vi "CG test stand DAQ main V2 variablized.vi"() -> ()   [LabVIEW 2020]
doc: "This example demonstrates how to read N channels of analog input from a LINX device."
uses:
  <vilib>/MakerHub/LINX/Public/Peripherals/Analog/Analog Read N Chans.vi
  <vilib>/MakerHub/LINX/Private/Local IO/LinxAnalogRead.vi
  <vilib>/MakerHub/LINX/Public/Utilities/Check Channel.vi
  <vilib>/MakerHub/LINX/Public/Utilities/Open Serial.vi
  <vilib>/MakerHub/LINX/Private/Utilties/Generate Error.vi
  <vilib>/Analysis/Matrix/Numeric/Conversions/Array To Matrix - RA.vi
  <vilib>/Utility/file.llb/Write Delimited Spreadsheet (DBL).vi
  <vilib>/MakerHub/LINX/LMH-LINX.lvlib
  <vilib>/Analysis/Matrix/NI_Matrix.lvlib
panel:
  in  "?":T1(tab)
  out "A8_Scaled":dbl
  out "A7_Scaled":dbl
  out "A6_Scaled":dbl
  out "C1 8":dbl
  out "C2 8":dbl
  out "C3 8":dbl
  out "B 8":dbl
  out "C1 7":dbl
  out "C2 7":dbl
  out "C3 7":dbl
  out "B 7":dbl
  out "C1 6":dbl
  out "C2 6":dbl
  out "C3 6":dbl
  out "B 6":dbl
  out "C1 5":dbl
  out "C2 5":dbl
  out "C3 5":dbl
  out "B 5":dbl
  out "C1 4":dbl
  out "C2 4":dbl
  out "C3 4":dbl
  out "B 4":dbl
  out "C1 3":dbl
  out "C2 3":dbl
  out "C3 3":dbl
  out "B 3":dbl
  out "C1 2":dbl
  out "C2 2":dbl
  out "C3 2":dbl
  out "B 2":dbl
  out "C1 1":dbl
  out "C2 1":dbl
  out "C3 1":dbl
  out "B 1":dbl
  out "C1 0":dbl
  out "C2 0":dbl
  out "C3 0":dbl
  out "B 0":dbl
  out "A0_Scaled":dbl
  out "A1_Instrumentlabel":string
  out "A8_Voltage":dbl
  out "A8":dbl
  out "A7_Voltage":dbl
  out "A7":dbl
  out "A6_Voltage":dbl
  out "A6":dbl
  out "A5_Voltage":dbl
  out "A5":dbl
  out "A4_Voltage":dbl
  out "A4":dbl
  out "A3_Voltage":dbl
  out "A3":dbl
  out "A2_Voltage":dbl
  out "A2":dbl
  out "A1_Voltage":dbl
  out "A1":dbl
  out "A0_Voltage":dbl
  out "A0_Instrumentlabel":dbl
  out "A2_Instrumentlabel":string
  out "A3_Instrumentlabel":string
  out "A4_Instrumentlabel":string
  out "A5_Instrumentlabel":string
  out "A6_Instrumentlabel":string
  out "A7_Instrumentlabel":string
  out "A8_Instrumentlabel":string
  out "A0_Instrumentlabel 2":string
  out "A1_Scaled":dbl
  out "A2_Scaled":dbl
  out "A3_Scaled":dbl
  out "A4_Scaled":dbl
  out "A5_Scaled":dbl
  in  "+      B":dbl
  in  "AX":dbl
  in  "Analog Port":dbl
  out "Time Stamp":timestamp
  out "Voltage":dbl
  out "Voltage":dbl(graph)
  out "Filtered Voltage":dbl(graph)
  out "Unfiltered Voltage":dbl
  out "Filtered Voltage":dbl
  out "?":dbl
  out "?":dbl
  out "?":dbl
  out "Orifice Temperature":dbl(knob) scale=0.0..10.0
  out "Reg Temperature":dbl(knob) scale=0.0..10.0
  out "Tank Temperature":dbl(knob) scale=0.0..10.0
  out "Temperatures":dbl[](graph)
  out "Orifice Pressure":dbl(knob) scale=0.0..10.0
  out "Reg Pressure":dbl(knob) scale=0.0..10.0
  out "Pressures":dbl[](graph)
  out "Tank Pressure":dbl(knob) scale=0.0..100.0
  in  "?":bool
  in  "Limited Rate (Hz)":dbl
  in  "?":bool
  out "Loop Rate (Hz)":u32
  in  "Stop Button":bool
  out "WRITING TO FILE":bool
  out "error out":errorcluster
  out "Full filepath":string
  in  "Path":path
  in  "File extension":string
  in  "Filename":string
  in  "Serial Port":refnum<visa-resource-name>
  # "Analog Inputs"
  # "Analog Port"
  # "Voltage In"
  # "X3"
  # "X2"
  # "X1"
  # "B"
  # "Instrument name"
  # "Scaled Value"
  # "File I/O"
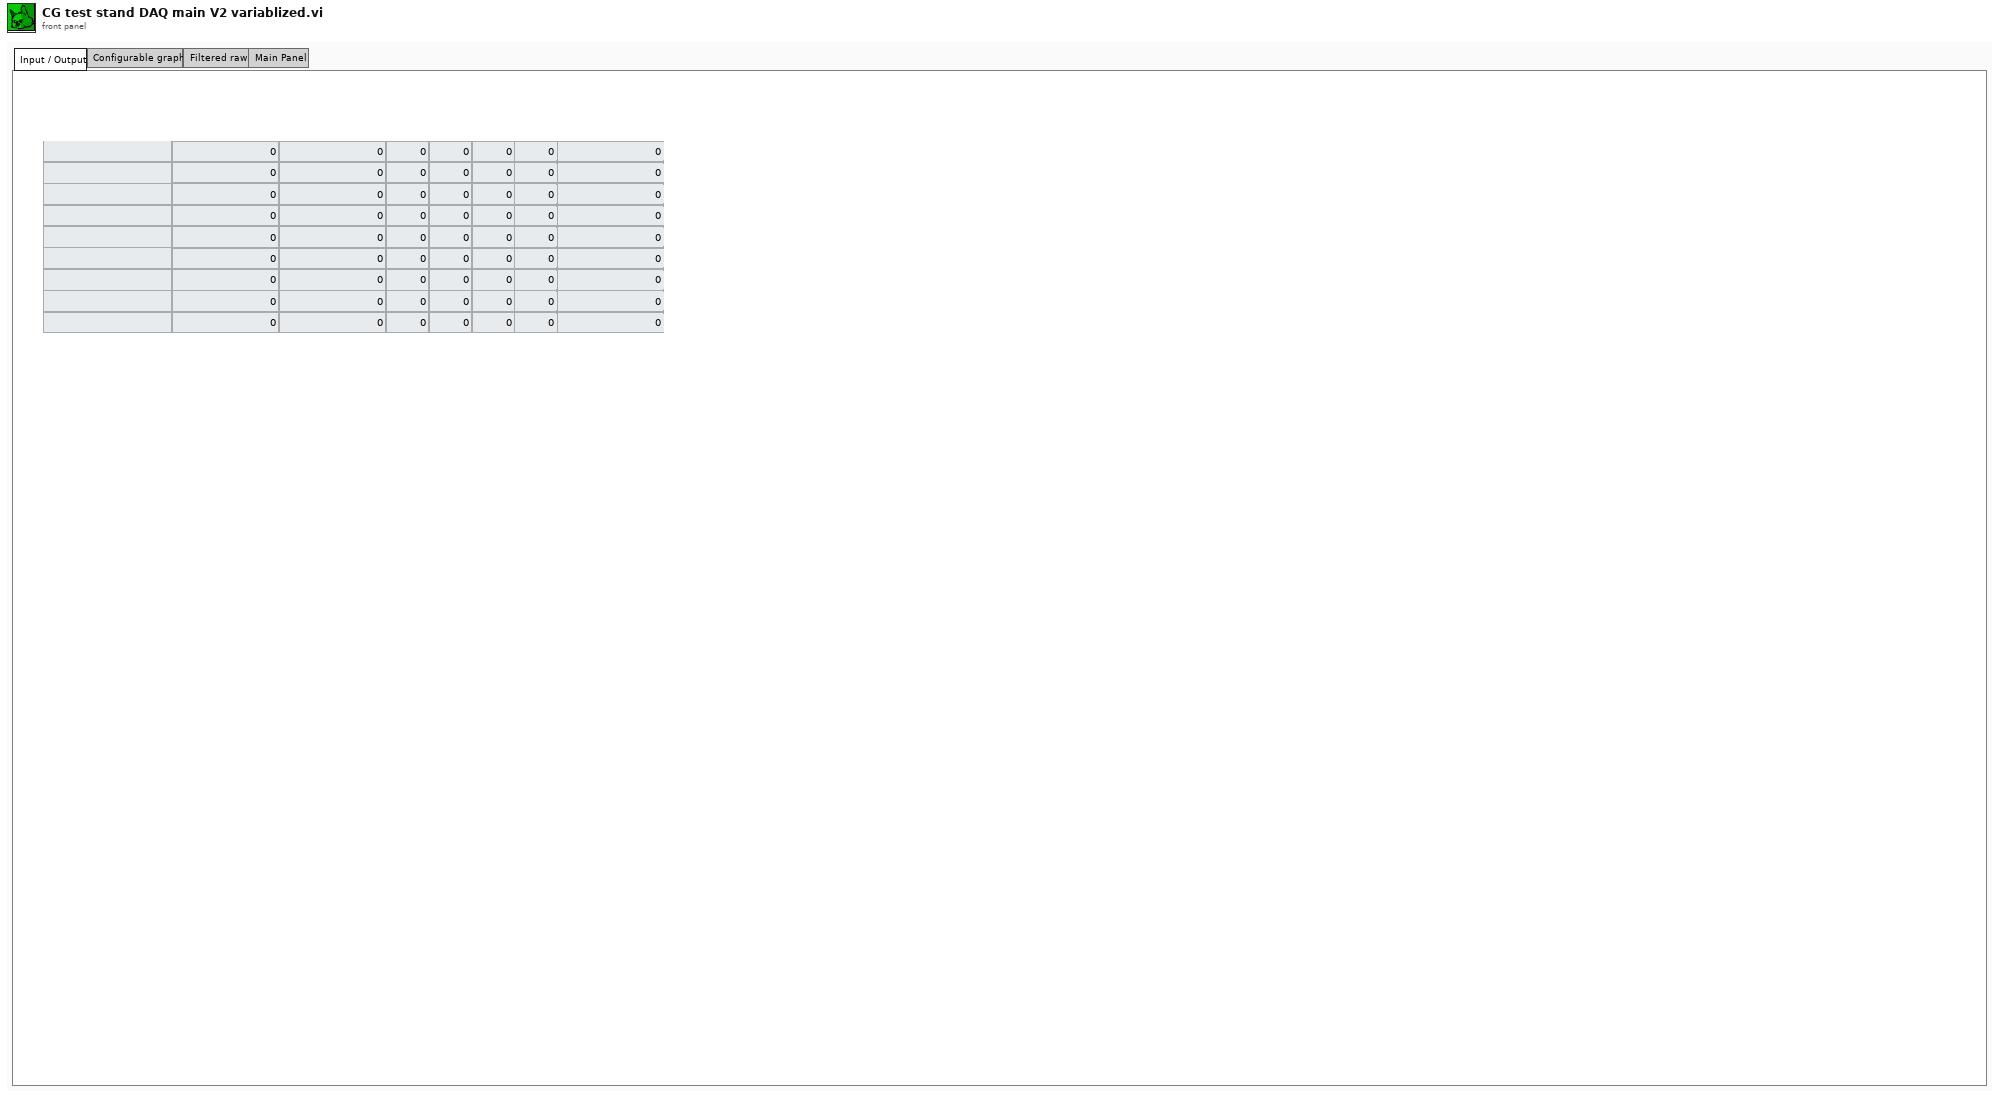
[diagram p1: front panel]
types:
  T1 = enum32{"Input / Output", "Configurable graph", "Filtered raw", "Main Panel"}
  T2 = typedef "LMH-LINX.lvlib/LINX Ref.ctl" = cluster{"IO":T3, "Interface":T4, "LINX Device Config":T5}
  T3 = typedef "LMH-LINX.lvlib/Platform.ctl" = enum16{"Remote", "Local"}
  T4 = typedef "LMH-LINX.lvlib/Interface.ctl" = enum16{"Serial", "TCP"}
  T5 = typedef "LMH-LINX.lvlib/Device.lvlib/LINX Device Config.ctl" = cluster{"Interface":T4, "COM Port":refnum<visa-resource-name>, "TCP Configuration":T6, "Device Family":u8, "Device ID":u8, "Device Name":string, "TCP Ref":refnum<k5>, "Channels":T7}
  T6 = typedef "LMH-LINX.lvlib/Device.lvlib/TCP Config.ctl" = cluster{"IP Address":string, "Port":u16}
  T7 = typedef "LMH-LINX.lvlib/Channels.ctl" = cluster{"DI":u8[], "DO":u8[], "AI":u8[], "AO":u8[], "PWM":u8[], "QE":u8[], "UART":u8[], "I2C 2":u8[], "SPI":u8[], "CAN":u8[], "Servo":u8[], "AI Ref (V)":dbl, "AI Resolution (Bits)":u8, "AO Ref (V)":dbl, "AO Resolution (Bits)":u8}
  T8 = typedef "NI_Matrix.lvlib/RealMatrix.ctl" = dbl[][]
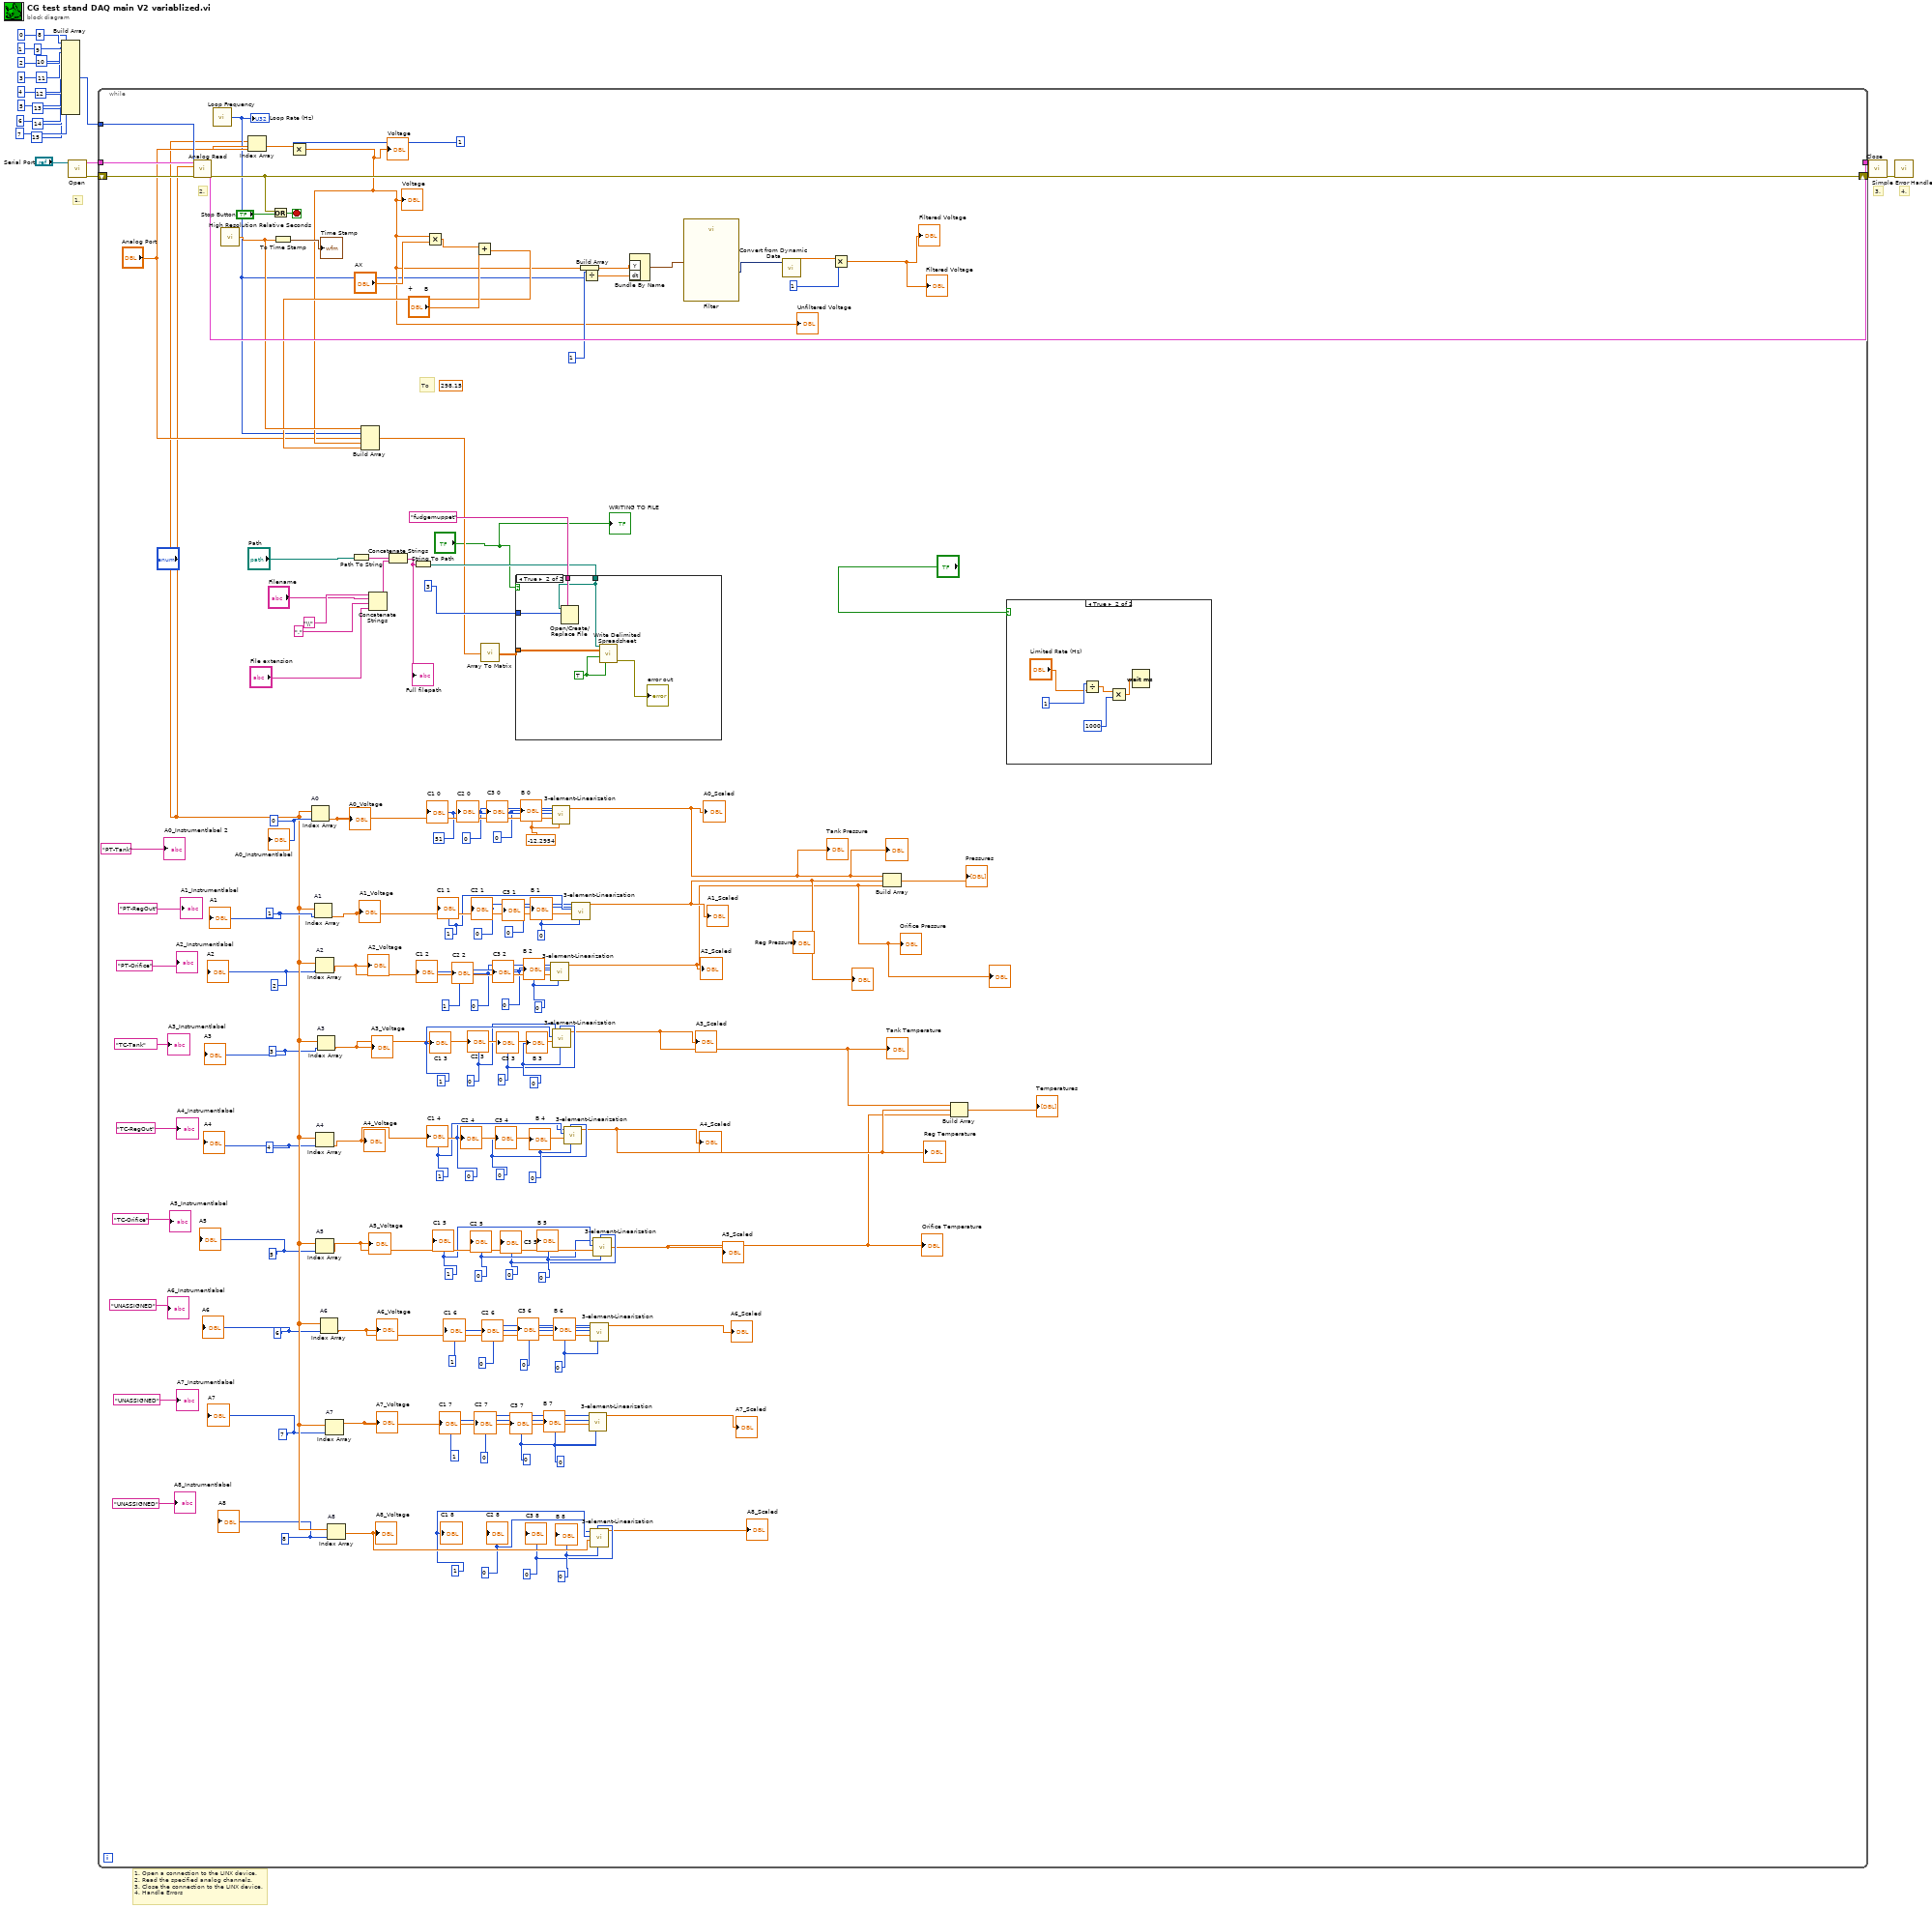
[diagram p0: block diagram]
diagram:
  # "1. Open a connection to the LINX device.\n2. Read the specified analog channels.\n3. Close the connection to the LINX device.\n4. Handle Errors"
  # "4."
  # "3."
  # "1."
  n1 = Build Array(0, 1, 2, 3, 4, 5, 6, 7, 8, 9, 10, 11, 12, 13, 14, 15) -> (w17:i32[])
  n2 = call-poly <vilib>:"Open.vi"("Serial Port"="Serial Port") -> ("Error Out"=w22:errorcluster, "LINX Resource"=w23:T2)  [unwired: 8 in, 1 out]
  n3 = while {
    tunnel: w23 -> [w139]
    tunnel: [w137] -> w21
    shift-right: [w134] -> w20
    shift-left: w22 -> [w138]
    tunnel: w17 -> [w133]
    stop <- w136 stop-if-true
    w42 = 0
    w39 = 0
    w40 = 0
    w41 = 1
    w48 = 0
    w45 = 0
    w46 = 0
    w47 = 1
    w54 = 0
    w51 = 0
    w52 = 0
    w53 = 1
    w37 = 0
    w34 = 0
    w35 = 0
    w36 = 1
    w60 = 0
    w57 = 0
    w58 = 0
    w59 = 1
    w65 = 0
    w62 = 0
    w63 = 0
    w64 = 1
    w69 = 0
    w66 = 0
    w67 = 0
    w68 = 1
    w73 = 0
    w70 = 0
    w71 = 0
    w72 = 1
    w77 = -12.2954
    w74 = 0
    w75 = 0
    w76 = 51
    w91 = 8
    w92 = 7
    w93 = 6
    w94 = 5
    w95 = 4
    w97 = 3
    w96 = 2
    w99 = 1
    w100 = 0
    (unwired) 298.15
    # "To"
    # "2."
    n4 = call-poly <vilib>:"Analog Read.vi"("Error In"=w138, "AI Channel(s)"=w133, "LINX Resource"=w139) -> ("Error Out"=w134:errorcluster, "Voltages"=w98:dbl[], "LINX Resource"=w137:T2)  [unwired: 5 in, 1 out]
    n5 = call <vilib>:"Loop Frequency.vi"() -> ("Loop Rate (Hz)"=w114:u32)
    "Loop Rate (Hz)" <- w114
    n6 = call <vilib>:"High Resolution Relative Seconds.vi"() -> ("relative seconds"=w128:dbl)
    n7 = Index Array(array=w98, index="Analog Port") -> (element=w123:dbl)
    n8 = Or(x=w134, y="Stop Button") -> (x .or. y?=w136:bool)
    n9 = To Time Stamp(1:w128) -> (0:→"Time Stamp":timestamp)
    n10 = Multiply(x=w123, y=1) -> (x*y=w116:dbl)
    "Voltage" <- w116
    "Voltage" <- w116
    "Unfiltered Voltage" <- w116
    n11 = Index Array "A0"(array=w98, index=w100) -> (element=w80:dbl)
    "A0_Voltage" <- w80
    n12 = Index Array "A1"(array=w98, index=w99) -> (element=w81:dbl)
    "A1_Voltage" <- w81
    n13 = Index Array "A2"(array=w98, index=w96) -> (element=w79:dbl)
    "A2_Voltage" <- w79
    n14 = Index Array "A4"(array=w98, index=w95) -> (element=w61:dbl)
    "A4_Voltage" <- w61
    n15 = Index Array "A5"(array=w98, index=w94) -> (element=w56:dbl)
    "A5_Voltage" <- w56
    n16 = Index Array "A3"(array=w98, index=w97) -> (element=w78:dbl)
    "A3_Voltage" <- w78
    n17 = Index Array "A6"(array=w98, index=w93) -> (element=w55:dbl)
    "A6_Voltage" <- w55
    n18 = Index Array "A7"(array=w98, index=w92) -> (element=w49:dbl)
    "A7_Voltage" <- w49
    n19 = Index Array "A8"(array=w98, index=w91) -> (element=w43:dbl)
    "A8_Voltage" <- w43
    n20 = Path To String(path="Path") -> (string=w108:string)
    n21 = Concatenate Strings("\\", "Filename", ".", "File extension") -> (w101:string)
    n22 = Concatenate Strings(w108, w101) -> (w109:string)
    "Full filepath" <- w109
    n23 = String To Path(string=w109) -> (path=w110:path)
    n24 = Multiply(x=w116, y="AX") -> (x*y=w130:dbl)
    n25 = Add(x=w130, y="+      B") -> (x+y=w117:dbl)
    n26 = Build Array(w128, w114, "Analog Port", w116, w117) -> (w106:dbl[])
    n27 = call-poly <vilib>:"Array To Matrix.vi"("Real 1D Array"=w106) -> ("Real Matrix (Column Vector)"=w113:T8)
    n28 = case shown="True" "?" {
      tunnel: w110 -> [_ w148]
      tunnel: w113 -> [_ w145]
      tunnel: "fudgemuppet" -> [_ w150]
      tunnel: 3 -> [_ w149]
      frame False {
      }
      frame True {
        w146 = TRUE
        n29 = Open/Create/Replace File(file path (use dialog)=w148, prompt=w150, operation (0:open)=w149) -> ()  [unwired: 3 in, 3 out]
        n30 = call-poly <vilib>:"Write Delimited Spreadsheet.vi"("file path (dialog if empty)"=w148, "2D data"=w145, "append to file? (new file:F)"=w146, "transpose? (no:F)"=w146) -> ("error out"=→"error out":errorcluster)  [unwired: 10 in, 1 out]
      }
    }
    n31 = call "3-element-Linearization.vi"("B"=w69, "C3"=w66, "Voltage in"=w79, "C1"=w68, "C2"=w67) -> ("Scaled value"=w24:dbl)  [unwired: 6 in]
    "A2_Scaled" <- w24
    "Orifice Pressure" <- w24
    "?" <- w24
    n32 = call "3-element-Linearization.vi"("B"=w77, "C3"=w74, "Voltage in"=w80, "C1"=w76, "C2"=w75) -> ("Scaled value"=w26:dbl)  [unwired: 6 in]
    "A0_Scaled" <- w26
    "Tank Pressure" <- w26
    "?" <- w26
    n33 = call "3-element-Linearization.vi"("B"=w65, "C3"=w62, "Voltage in"=w78, "C1"=w64, "C2"=w63) -> ("Scaled value"=w30:dbl)  [unwired: 6 in]
    "A3_Scaled" <- w30
    "Tank Temperature" <- w30
    n34 = call "3-element-Linearization.vi"("B"=w60, "C3"=w57, "Voltage in"=w61, "C1"=w59, "C2"=w58) -> ("Scaled value"=w29:dbl)  [unwired: 6 in]
    "A4_Scaled" <- w29
    "Reg Temperature" <- w29
    n35 = call "3-element-Linearization.vi"("B"=w73, "C3"=w70, "Voltage in"=w81, "C1"=w72, "C2"=w71) -> ("Scaled value"=w25:dbl)  [unwired: 6 in]
    "A1_Scaled" <- w25
    "Reg Pressure" <- w25
    "?" <- w25
    n36 = Build Array(w116) -> (w125:dbl[])
    n37 = Divide(x=1, y=w114) -> (x/y=w127:dbl)
    n38 = call "3-element-Linearization.vi"("B"=w48, "C3"=w45, "Voltage in"=w49, "C1"=w47, "C2"=w46) -> ("Scaled value"=→"A7_Scaled":dbl)  [unwired: 6 in]
    n39 = call "3-element-Linearization.vi"("B"=w54, "C3"=w51, "Voltage in"=w55, "C1"=w53, "C2"=w52) -> ("Scaled value"=→"A6_Scaled":dbl)  [unwired: 6 in]
    n40 = call "3-element-Linearization.vi"("B"=w42, "C3"=w39, "Voltage in"=w43, "C1"=w41, "C2"=w40) -> ("Scaled value"=→"A8_Scaled":dbl)  [unwired: 6 in]
    n41 = call "3-element-Linearization.vi"("B"=w37, "C3"=w34, "Voltage in"=w56, "C1"=w36, "C2"=w35) -> ("Scaled value"=w28:dbl)  [unwired: 6 in]
    "A5_Scaled" <- w28
    "Orifice Temperature" <- w28
    n42 = Bundle By Name("Y"=w125, "dt"=w127) -> (w124:waveform(dbl))  [unwired: 1 in]
    n43 = call "Filter"("Signal"=w124) -> ("Filtered Signal"=w121:dynamicdata)  [unwired: 9 in, 1 out]
    n44 = call "Convert from Dynamic Data"("Dynamic Data Type"=w121) -> ("Scalar"=w120:dbl)  [unwired: 3 in]
    n45 = Multiply(x=w120, y=1) -> (x*y=→"Filtered Voltage" →"Filtered Voltage":dbl)
    n46 = Build Array(w26, w25, w24) -> (→"Pressures":dbl[])
    n47 = Build Array(w30, w29, w28) -> (→"Temperatures":dbl[])
    n48 = case shown="True" "?" {
      frame False {
      }
      frame True {
        n49 = Divide(x=1, y="Limited Rate (Hz)") -> (x/y=w141:dbl)
        n50 = Multiply(x=w141, y=1000) -> (x*y=w140:dbl)
        n51 = Wait (ms)(milliseconds to wait=w140) -> ()  [unwired: 1 out]
      }
    }
    "WRITING TO FILE" <- "?"
    "A0_Instrumentlabel" <- w100
    "A1" <- w99
    "A2" <- w96
    "A3" <- w97
    "A4" <- w95
    "A5" <- w94
    "A6" <- w93
    "A7" <- w92
    "A8" <- w91
    "A1_Instrumentlabel" <- "PT-RegOut"
    "A2_Instrumentlabel" <- "PT-Orifice"
    "A3_Instrumentlabel" <- "TC-Tank"
    "A4_Instrumentlabel" <- "TC-RegOut"
    "A5_Instrumentlabel" <- "TC-Orifice"
    "A6_Instrumentlabel" <- "UNASSIGNED"
    "A7_Instrumentlabel" <- "UNASSIGNED"
    "A8_Instrumentlabel" <- "UNASSIGNED"
    "A0_Instrumentlabel 2" <- "PT-Tank"
    "B 0" <- w77
    "C3 0" <- w74
    "C2 0" <- w75
    "C1 0" <- w76
    "B 1" <- w73
    "C3 1" <- w70
    "C2 1" <- w71
    "C1 1" <- w72
    "B 2" <- w69
    "C3 2" <- w66
    "C2 2" <- w67
    "C1 2" <- w68
    "B 3" <- w65
    "C3 3" <- w62
    "C2 3" <- w63
    "C1 3" <- w64
    "B 4" <- w60
    "C3 4" <- w57
    "C2 4" <- w58
    "C1 4" <- w59
    "B 5" <- w37
    "C3 5" <- w34
    "C2 5" <- w35
    "C1 5" <- w36
    "B 6" <- w54
    "C3 6" <- w51
    "C2 6" <- w52
    "C1 6" <- w53
    "B 7" <- w48
    "C3 7" <- w45
    "C2 7" <- w46
    "C1 7" <- w47
    "B 8" <- w42
    "C3 8" <- w39
    "C2 8" <- w40
    "C1 8" <- w41
  }
  n52 = call <vilib>:"Close.vi"("Error In"=w20, "LINX Resource"=w21) -> ("Error Out"=w18:errorcluster)  [unwired: 9 in]
  n53 = call <vilib>:"Simple Error Handler.vi"("error in (no error)"=w18) -> ()  [unwired: 4 in, 5 out]
